vi "Write Error to System Log.vi"(8 "error in":errorcluster, 11 "execution unit identifier":string="custom device") -> (0 "error out":errorcluster)   [LabVIEW 2020, in "Ballard ARINC 429 Engine.lvlib" / "Custom Device.lvlib"]
uses:
  Custom Device.lvlib
  <vilib>/NI VeriStand/Custom Device Tools/Custom Device Utility Library/Custom Device Utility Library.lvlib
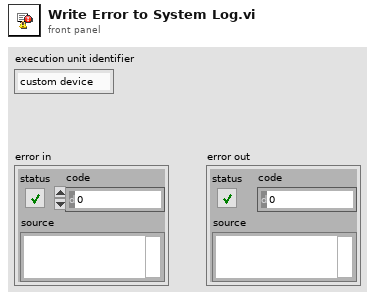
[diagram p1: front panel]
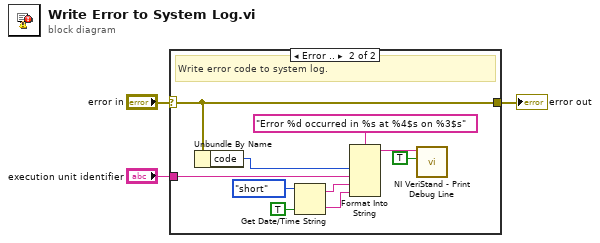
[diagram p0: block diagram]
diagram:
  n1 = case shown="Error .." "error in" {
    selector: "error in" -> [w4 w14]
    tunnel: [w4 w14] -> w3
    tunnel: "execution unit identifier" -> [_ w12]
    frame No Error {
      # "Do not log OK - this is not a heartbeat.\nDo not log warnings."
    }
    frame Error {
      # "Write error code to system log."
      n2 = Unbundle By Name(w14) -> ("code"=w13:i32)
      n3 = Get Date/Time String(date format (0)=enum16{"short", "long", "abbreviated"}."short", want seconds? (F)=TRUE) -> (date string=w9:string, time string=w8:string)  [unwired: 1 in]
      n4 = Format Into String(format string="Error %d occurred in %s at %4$s on %3$s", w13, w12, w9, w8) -> (resulting string=w10:string)  [unwired: 2 in, 1 out]
      n5 = call <vilib>:"NI VeriStand - Print Debug Line.vi"("Add to log file? (F)"=TRUE, "Message"=w10) -> ()  [unwired: 9 in, 1 out]
    }
  }
  "error out" <- w3
